vi "Create.vi"() -> (7 "Historian Charting Manager ID out":refnum<class "Historian Charting Manager ID.lvclass">)   [LabVIEW 2020, in "VolatusGUI.lvlib" / "Historian Charting Manager ID.lvclass"]
uses:
  Historian Charting Manager ID.lvclass
  Historian Charting Manager ID.lvclass/Historian Charting Manager ID.ctl
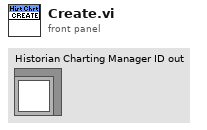
[diagram p1: front panel]
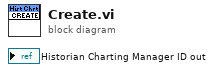
[diagram p0: block diagram]
diagram:
